vi "Convert Double Precision.vi"(10 "Input":dbl) -> (2 "Output":dbl)   [LabVIEW 2018]
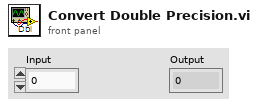
[diagram p1: front panel]
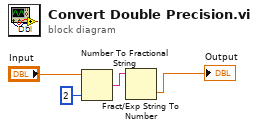
[diagram p0: block diagram]
diagram:
  n1 = Number To Fractional String(number="Input", precision (6)=i16 2) -> (F-format string=w2:string)  [unwired: 2 in]
  n2 = Fract/Exp String To Number(string=w2) -> (number=→"Output":dbl)  [unwired: 3 in, 1 out]
